vi "Get Enum Values.vi"(11 "UI Data in":refnum<class "Settings UI.lvclass">) -> (1 "Enum Values":string[](array[string]), 2 "Default Value":string, 3 "UI Data out":refnum<class "Settings UI.lvclass">)   [LabVIEW 2020, in "Output Sequencer.lvlib" / "Settings UI.lvclass"]
uses:
  Settings UI.lvclass
  Settings UI.lvclass/Settings UI.ctl
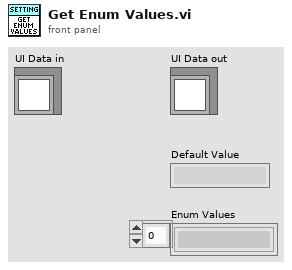
[diagram p1: front panel]
types:
  T1 = typedef "Output Sequencer.lvlib/Settings UI.lvclass/Step Settings.ctl" = cluster{"Description":string, "Precondition":string, "Duration":dbl, "Mode":string, "Delay Between Values":dbl, "Analog Values":string[], "Digital Values":string[], "Postcondition":string, "On True":string, "On False":string}
  T2 = typedef "Output Sequencer.lvlib/Settings UI.lvclass/Tree Item Settings.ctl" = cluster{"Tree Label":string, "Indent Level":i32, "Data Type":T3, "Numeric Range":cluster{"Min":dbl, "Max":dbl, "Inc":dbl}, "Allowed Values":string[], "Default Value":string, "Description":string}
  T3 = typedef "Output Sequencer.lvlib/Settings UI.lvclass/Data Type.ctl" = i16
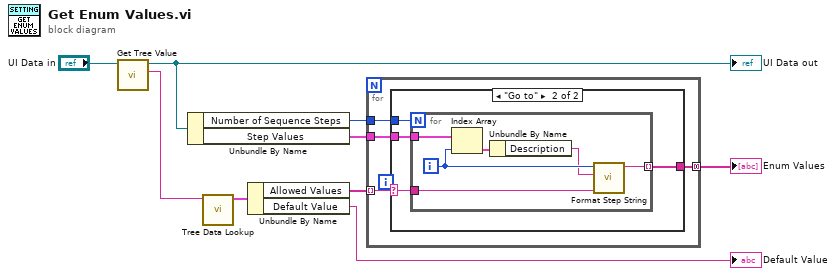
[diagram p0: block diagram]
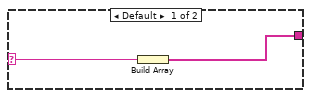
[diagram p2: hidden frame]
diagram:
  n1 = call "Get Tree Value.vi"("UI Data in"="UI Data in") -> ("Value"=w3:string, "UI Data out"=w7:refnum<class "Settings UI.lvclass">)  [unwired: 9 in]
  "UI Data out" <- w7
  n2 = Unbundle By Name(w7) -> ("Number of Sequence Steps"=w2:i32, "Step Values"=w1:T1[])
  n3 = call "Tree Data Lookup.vi"("Tag in"=w3) -> ("Tree Data"=w4:T2)  [unwired: 5 in, 5 out]
  n4 = Unbundle By Name(w4) -> ("Allowed Values"=w5:string[], "Default Value"=→"Default Value":string)
  n5 = for {
    tunnel: [w13] -> w8 mode=concatenating
    tunnel: w5 -> [w12] mode=indexing
    tunnel: w2 -> [w11]
    tunnel: w1 -> [w10]
    n6 = case shown="\"Go to\"" w12 {
      selector: w12 -> [w15 w18]
      tunnel: [w14 w19] -> w13
      tunnel: w11 -> [_ w17]
      tunnel: w10 -> [_ w16]
      frame Default {
        n7 = Build Array(w15) -> (w14:string[])
      }
      frame "Go to" {
        n8 = for {
          N: w17 -> [_]
          tunnel: w18 -> [w25]
          tunnel: [w24] -> w19 mode=indexing
          tunnel: w16 -> [w23]
          i -> [w22]
          n9 = Index Array(array=w23, index=w22) -> (element=w21:T1)
          n10 = Unbundle By Name(w21) -> ("Description"=w20:string)
          n11 = call "Format Step String.vi"("Initial string (default: \"Step\")"=w25, "Description"=w20, "Step Number"=w22) -> ("String"=w24:string)  [unwired: 8 in]
        }
      }
    }
  }
  "Enum Values" <- w8
